vi "Notify.vi"(8 "error in (no error)":errorcluster, 11 "CS++SVMonitor in":refnum<class "CS++SVMonitor.lvclass">) -> (0 "error out":errorcluster, 3 "CS++SVMonitor out":refnum<class "CS++SVMonitor.lvclass">)   [LabVIEW 2012, in "CS++SVMonitor.lvlib" / "CS++SVMonitor.lvclass"]
doc: "Notify PV readout."
uses:
  CS++SVMonitor.lvclass
  CS++PVMonitor/CS++PVMonitor.lvclass/CS++PVMonitor.ctl
  CS++SVMonitor.lvclass/CS++SVMonitor.ctl
  <vilib>/ActorFramework/Message Enqueuer/Message Enqueuer.lvclass
  CS++PVMonitor Messages/CS++PVUpdate Msg/CS++PVUpdate Msg.lvclass
  CS++PVMonitor/CS++PVMonitor.lvclass
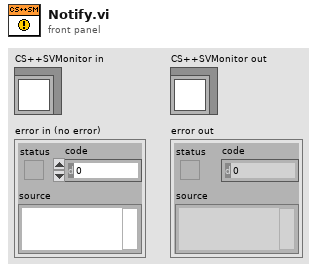
[diagram p1: front panel]
types:
  T1 = cluster{"PV URL":string, "Observers":cluster{"Enqueuer":refnum<class "Message Enqueuer.lvclass">, "CS++PVUpdate Msg":refnum<class "CS++PVUpdate Msg.lvclass">}[]}[]
  T2 = cluster{"SV Refnums":refnum<k21>[], "PV Connections":cluster{"PV URL":string, "Observers":cluster{"Enqueuer":refnum<class "Message Enqueuer.lvclass">, "CS++PVUpdate Msg":refnum<class "CS++PVUpdate Msg.lvclass">}[]}[]}
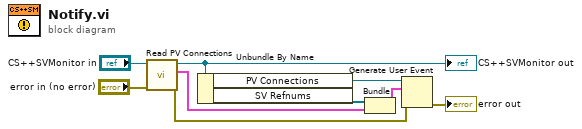
[diagram p0: block diagram]
diagram:
  n1 = call "Read PV Connections.vi"("error in (no error)"="error in (no error)", "CS++PVMonitor in"="CS++SVMonitor in") -> ("error out"=w2:errorcluster, "PV Connections"=w6:T1, "CS++PVMonitor out"=w5:refnum<class "CS++SVMonitor.lvclass">)  [unwired: 7 in]
  "CS++SVMonitor out" <- w5
  n2 = Unbundle By Name(w5) -> ("PV Connections"=w4:refnum<user-event>, "SV Refnums"=w7:refnum<k21>[])
  n3 = Bundle("SV Refnums"=w7, "PV Connections"=w6) -> (w3:T2)  [unwired: 1 in]
  n4 = Generate User Event(user event=w4, event data cluster=w3, error in=w2) -> (error out=→"error out":errorcluster)  [unwired: 1 out]
